vi "my_GPIB_comm_IPS.vi"(2 "error in":errorcluster, 3 "Command":string, 4 "Timeout (ms)":u32, 5 "GPIB address":string) -> (0 "error out":errorcluster, 1 "Reply from Instrument":string)   [LabVIEW 2025, in "Cryo.lvlib"]
uses:
  Cryo.lvlib
panel:
  in  "Case Constant\n(See Context Help) 2":bool=TRUE
  in  "Case Constant\n(See Context Help)":bool=TRUE
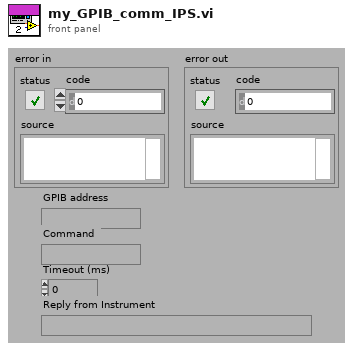
[diagram p1: front panel]
types:
  T1 = enum16{"Initialise GPIB", "Clear Device", "Read Serial Poll if Necessary", "Write \"V\" for version command of instrument", "If \"write\" successful, wait for Serial Poll", "\"Read\" reply", "Read the Serial Poll", "Exit"}
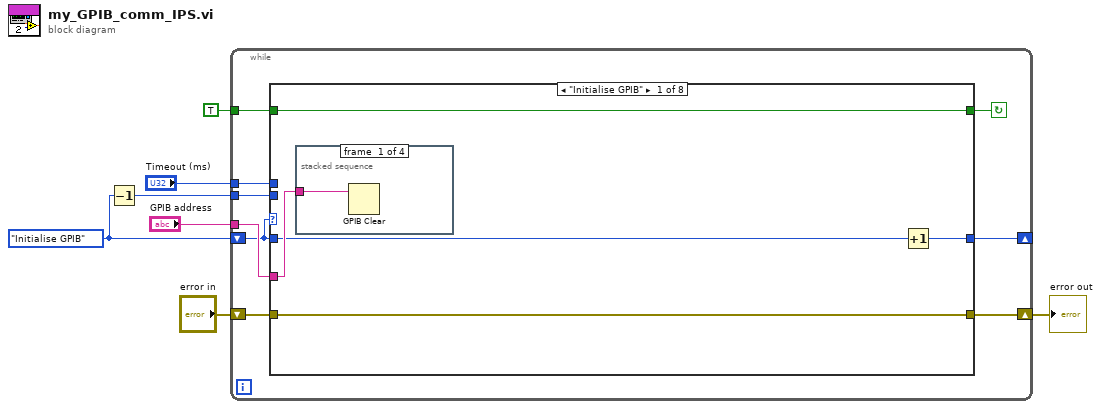
[diagram p0: block diagram]
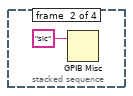
[diagram p2: hidden frame]
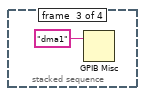
[diagram p3: hidden frame]
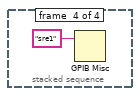
[diagram p4: hidden frame]
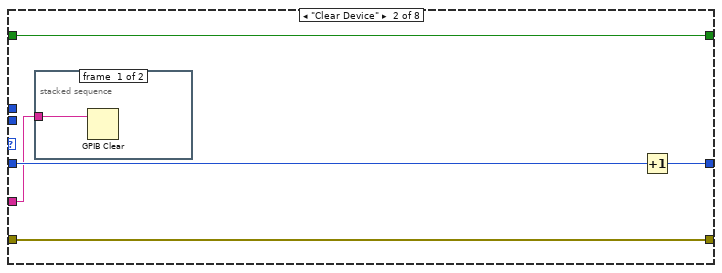
[diagram p5: hidden frame]
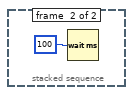
[diagram p6: hidden frame]
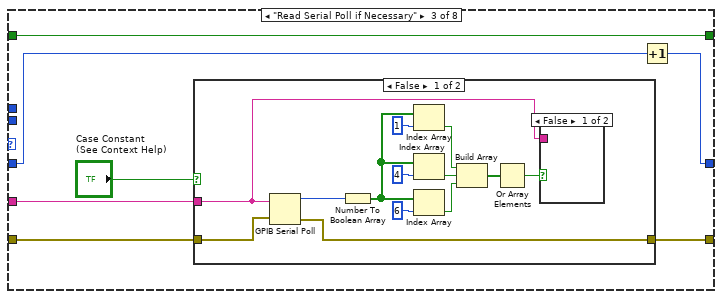
[diagram p7: hidden frame]
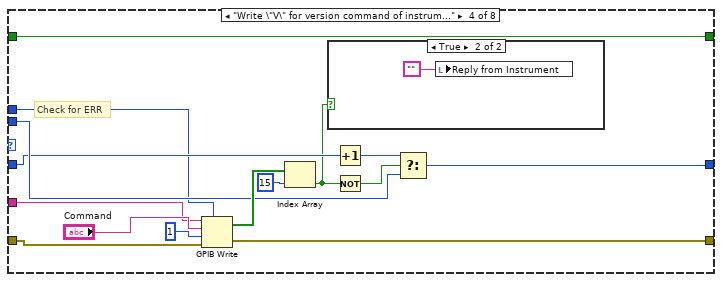
[diagram p10: hidden frame]
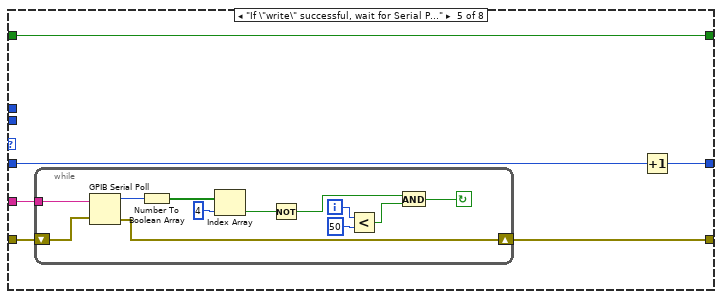
[diagram p12: hidden frame]
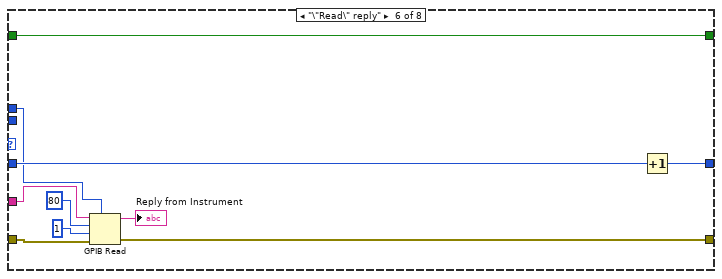
[diagram p13: hidden frame]
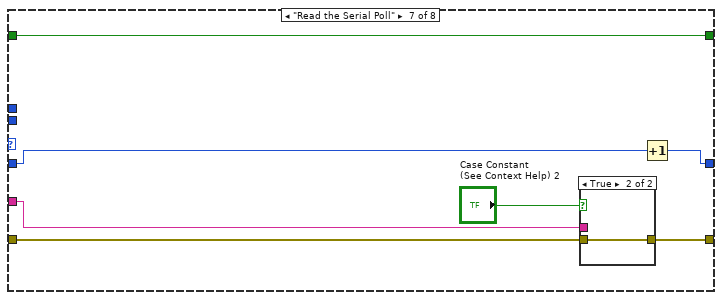
[diagram p14: hidden frame]
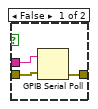
[diagram p15: hidden frame]
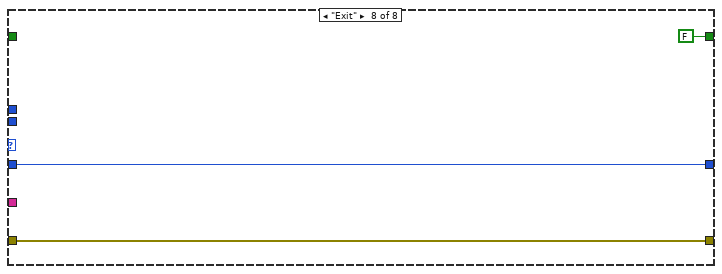
[diagram p16: hidden frame]
diagram:
  w6 = T1."Initialise GPIB"
  n1 = Decrement(x=w6) -> (x-1=w7:T1)
  n2 = while {
    tunnel: "Timeout (ms)" -> [w10]
    shift-left: w6 -> [w11]
    shift-right: [w12] -> _
    tunnel: TRUE -> [w13]
    tunnel: "GPIB address" -> [w15]
    tunnel: w7 -> [w16]
    shift-right: [w9] -> w1
    shift-left: "error in" -> [w8]
    stop <- w14 continue-if-true
    n3 = case shown="\"Initialise GPIB\"" w11 {
      tunnel: w15 -> [w21 w27 w39 w56 w75 w96 w104 _]
      tunnel: [w19 w29 w36 w63 w73 w93 w102 w111] -> w12
      tunnel: w11 -> [w20 w30 w37 w64 w74 w94 w103 w111]
      tunnel: w16 -> [_ _ _ w65 _ _ _ _]
      tunnel: [w18 w28 w35 w60 w72 w92 w101 FALSE] -> w14
      tunnel: w13 -> [w18 w28 w35 w60 w72 w92 w101 _]
      tunnel: w10 -> [_ _ _ w57 _ w90 _ _]
      tunnel: [w17 w26 w33 w55 w70 w88 w98 w109] -> w9
      tunnel: w8 -> [w17 w26 w34 w54 w71 w89 w99 w109]
      frame "Initialise GPIB" {
        n4 = stacked-sequence {
          tunnel: w21 -> [w22 _ _ _]
          frame #0 {
            n5 = GPIB Clear(3:w22) -> ()  [unwired: 1 in, 2 out]
          }
          frame #1 {
            n6 = GPIB Misc(0:"sic") -> ()  [unwired: 1 in, 3 out]
          }
          frame #2 {
            n7 = GPIB Misc(0:"dma1") -> ()  [unwired: 1 in, 3 out]
          }
          frame #3 {
            n8 = GPIB Misc(0:"sre1") -> ()  [unwired: 1 in, 3 out]
          }
        }
        n9 = Increment(x=w20) -> (x+1=w19:T1)
      }
      frame "Clear Device" {
        n10 = stacked-sequence {
          tunnel: w27 -> [w31 _]
          frame #0 {
            n11 = GPIB Clear(3:w31) -> ()  [unwired: 1 in, 2 out]
          }
          frame #1 {
            n12 = Wait (ms)(milliseconds to wait=u32 100) -> ()  [unwired: 1 out]
          }
        }
        n13 = Increment(x=w30) -> (x+1=w29:T1)
      }
      frame "Read Serial Poll if Necessary" {
        n14 = case shown="False" "Case Constant\n(See Context Help)" {
          tunnel: w39 -> [w52 _]
          tunnel: w34 -> [w41 w53]
          tunnel: [w40 w53] -> w33
          frame False {
            n15 = GPIB Serial Poll(0:w52, 1:w41) -> (2:w42:i16, 4:w40:errorcluster)  [unwired: 1 out]
            n16 = Number To Boolean Array(number=w42) -> (Boolean array=w46:bool[])
            n17 = Index Array(array=w46, index=1) -> (element=w48:bool)
            n18 = Index Array(array=w46, index=4) -> (element=w47:bool)
            n19 = Index Array(array=w46, index=6) -> (element=w49:bool)
            n20 = Build Array(w48, w47, w49) -> (w50:bool[])
            n21 = Or Array Elements(Boolean array=w50) -> (logical OR=w51:bool)
            n22 = case shown="False" w51 {
              tunnel: w52 -> [_ _]
              frame False {
              }
              frame True {
              }
            }
          }
          frame True {
          }
        }
        n23 = Increment(x=w37) -> (x+1=w36:T1)
      }
      frame "Write \"V\" for version command of instrument" {
        # "Check for ERR"
        n24 = GPIB Write(0:w56, 1:"Command", 2:1, 3:w54, 4:w57) -> (5:w67:bool[], 6:w55:errorcluster)
        n25 = Index Array(array=w67, index=15) -> (element=w59:bool)
        n26 = case shown="True" w59 {
          frame False {
          }
          frame True {
            n27 = local write "Reply from Instrument"("") -> ()
          }
        }
        n28 = Increment(x=w64) -> (x+1=w61:T1)
        n29 = Not(x=w59) -> (.not. x?=w62:bool)
        n30 = Select(t=w61, s=w62, f=w65) -> (s? t:f=w63:T1)
      }
      frame "If \"write\" successful, wait for Serial Poll" {
        n31 = while {
          tunnel: w75 -> [w84]
          shift-right: [w76] -> w70
          shift-left: w71 -> [w77]
          i -> [w82]
          stop <- w78 continue-if-true
          n32 = GPIB Serial Poll(0:w84, 1:w77) -> (2:w85:i16, 4:w76:errorcluster)  [unwired: 1 out]
          n33 = Number To Boolean Array(number=w85) -> (Boolean array=w86:bool[])
          n34 = Index Array(array=w86, index=4) -> (element=w83:bool)
          n35 = Not(x=w83) -> (.not. x?=w80:bool)
          n36 = Less?(x=w82, y=50) -> (x < y?=w79:bool)
          n37 = And(x=w80, y=w79) -> (x .and. y?=w78:bool)
        }
        n38 = Increment(x=w74) -> (x+1=w73:T1)
      }
      frame "\"Read\" reply" {
        n39 = GPIB Read(0:w96, 1:80, 2:1, 3:w89, 4:w90) -> (5:→"Reply from Instrument":string, 7:w88:errorcluster)  [unwired: 1 out]
        n40 = Increment(x=w94) -> (x+1=w93:T1)
      }
      frame "Read the Serial Poll" {
        n41 = case shown="True" "Case Constant\n(See Context Help) 2" {
          tunnel: w104 -> [w107 _]
          tunnel: w99 -> [w106 w108]
          tunnel: [w105 w108] -> w98
          frame False {
            n42 = GPIB Serial Poll(0:w107, 1:w106) -> (4:w105:errorcluster)  [unwired: 2 out]
          }
          frame True {
          }
        }
        n43 = Increment(x=w103) -> (x+1=w102:T1)
      }
      frame "Exit" {
      }
    }
  }
  "error out" <- w1
